vi "Actor Core.vi"(8 "error in":errorcluster, 11 "Assembly Run in":refnum<class "Assembly Run.lvclass">) -> (0 "error out":errorcluster, 3 "Actor out":refnum<class "Actor.lvclass">)   [LabVIEW 2020, in "Assembly Run.lvclass"]
doc: "(<B>Filename</B>: Actor Framework.lvlib:Actor.lvclass:Actor Core.vi)\n\nReceives messages to the actor, reacts to them, and initiates any error handling that may shut the actor down.\n\nDescendant classes may override this VI to append parallel tasks for the actor to complete while it handles messages. Overrides use the Call Parent Class Method node."
uses:
  Assembly Run.lvclass
  <vilib>/ActorFramework/Actor/Actor.lvclass
  Workspace/Fixture.lvclass
  Routine/Routine.lvclass
  <vilib>/ActorFramework/Message Enqueuer/Message Enqueuer.lvclass
  C:/Program Files/National Instruments/LabVIEW 2020/vi.lib/ActorFramework/Actor/Actor.lvclass
  C:/Users/hep/Documents/CMU gantry/Classes/Assembly/Assembly Run.lvclass
  C:/Users/hep/Documents/CMU gantry/Classes/Workspace/Fixture.lvclass
  C:/Users/hep/Documents/CMU gantry/Classes/Routine/Routine.lvclass
  Routine/Routine Enum.ctl
  Workspace/Fixture Enum.ctl
panel:
  in  "Fixtures":T1[](array[typedef])
  in  "Routines":T2[](array[typedef])
  in  "run":bool
  in  "find centers":bool
  in  "add":bool
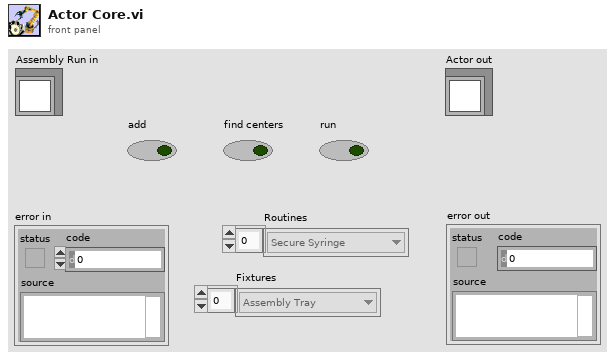
[diagram p1: front panel]
types:
  T1 = typedef "Fixture.lvclass/Fixture Enum.ctl" = enum16{"Assembly Tray", "Syringe Space", "Component", "Pick Up Tool", "Current Position"}
  T2 = typedef "Routine.lvclass/Routine Enum.ctl" = enum16{"Primary Pick Up", "Pick Up All", "Put Down Secondary", "Put Down All", "Release Syringe", "Secondary Pick Up", "Secure Syringe", "Dispense on Plate", "Dispense on Kapton", "Dispense on Sensor"}
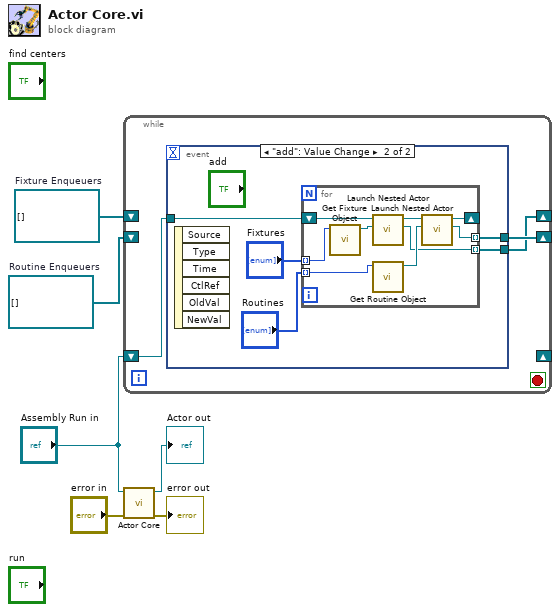
[diagram p0: block diagram]
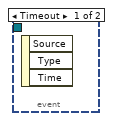
[diagram p2: hidden frame]
diagram:
  w1 = refnum<class "Message Enqueuer.lvclass">[] []  # Routine Enqueuers
  w2 = refnum<class "Message Enqueuer.lvclass">[] []  # Fixture Enqueuers
  n1 = while {
    shift-right: _ -> [_]
    shift-left: "Assembly Run in" -> [w9]
    shift-right: [w7] -> _
    shift-left: w2 -> [_]
    shift-right: [w8] -> _
    shift-left: w1 -> [_]
    stop <- _ stop-if-true
    n2 = event shown="[1] \"add\": Value Change" {
      selector: _ -> [_ _]
      dyn-events: _ -> [_ _]
      timeout: _ -> [_ _]
      tunnel: w9 -> [_ w12]
      tunnel: [_ w11] -> w8
      tunnel: [_ w10] -> w7
      event Timeout {
        n3 = event-data() -> ()  [unwired: 1 in, 3 out]
      }
      event "add": Value Change {
        n4 = event-data() -> ()  [unwired: 1 in, 6 out]
        n5 = for {
          tunnel: "Routines" -> [w23] mode=indexing
          tunnel: "Fixtures" -> [w22] mode=indexing
          shift-right: [w18] -> _
          shift-left: w12 -> [w20]
          tunnel: [w16] -> w10 mode=indexing
          tunnel: [w15] -> w11 mode=indexing
          n6 = call "Get Fixture Object.vi"("Fixture"=w22) -> ("Workspace.lvclass"=w21:refnum<class "Fixture.lvclass">)  [unwired: 8 in, 2 out]
          n7 = call <vilib>:"Launch Nested Actor.vi"("Nested Actor"=w21, "Caller Actor in"=w20) -> ("Nested Actor's Enqueuer"=w16:refnum<class "Message Enqueuer.lvclass">, "Caller Actor out"=w19:refnum<class "Assembly Run.lvclass">)  [unwired: 7 in, 1 out]
          n8 = call "Get Routine Object.vi"("Routine"=w23) -> ("Routine out"=w17:refnum<class "Routine.lvclass">)  [unwired: 9 in, 1 out]
          n9 = call <vilib>:"Launch Nested Actor.vi"("Nested Actor"=w17, "Caller Actor in"=w19) -> ("Nested Actor's Enqueuer"=w15:refnum<class "Message Enqueuer.lvclass">, "Caller Actor out"=w18:refnum<class "Assembly Run.lvclass">)  [unwired: 7 in, 1 out]
        }
      }
    }
  }
  n10 = call-parent "Actor Core.vi"("error in"="error in", "Actor in"="Assembly Run in") -> ("error out"=→"error out":errorcluster, "Actor out"=→"Actor out":refnum<class "Actor.lvclass">)  [unwired: 8 in]
